vi "TDMS_Waveform to file.vi"(0 "Base path":path, 1 "Group Name":string="A", 2 "Interval":T1=enum."Daily", 3 "UTC Time FPGA":u64[](array[numeric]), 5 "Measurement":string, 9 "element":waveform(dbl)[](array[waveform]), 11 "error in (no error)":errorcluster, 12 "Channel Names":string[](array[string]), 13 "property values":variant[](array[variant]), 14 "UTC Time SC":u64[](array[numeric])) -> (4 "file out":refnum<k34>, 15 "error out":errorcluster)   [LabVIEW 2019]
uses:
  Globals and Definitions/Enum_FileNewInterval.ctl
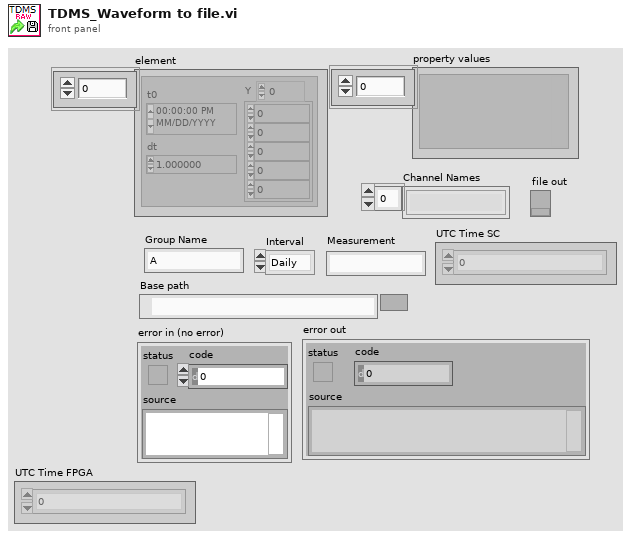
[diagram p1: front panel]
types:
  T1 = typedef "Enum_FileNewInterval.ctl" = enum16{"10 Min", "Hourly", "Daily", "Weekly", "Monthly"}
  T2 = enum16{"open", "open or create", "create or replace", "create", "open (read-only)"}
  T3 = typedef "LVDateTimeRec.ctl" = cluster{"fractional second":dbl, "second":i32, "minute":i32, "hour":i32, "day of month":i32, "month":i32, "year":i32, "day of week":i32, "day of year":i32, "DST":i32}
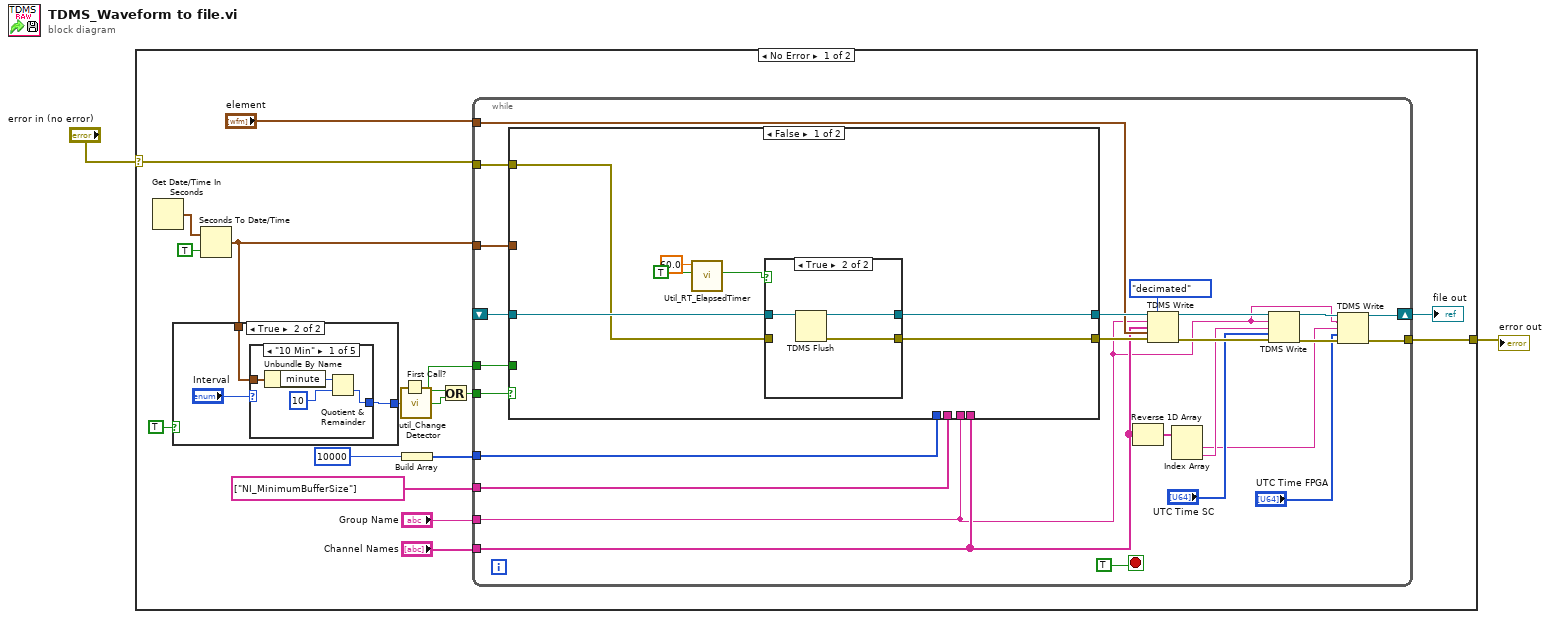
[diagram p0: block diagram]
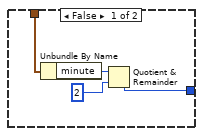
[diagram p2: hidden frame]
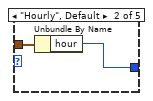
[diagram p3: hidden frame]
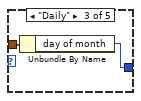
[diagram p4: hidden frame]
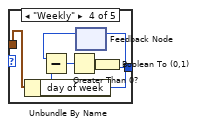
[diagram p5: hidden frame]
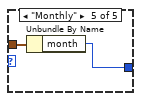
[diagram p6: hidden frame]
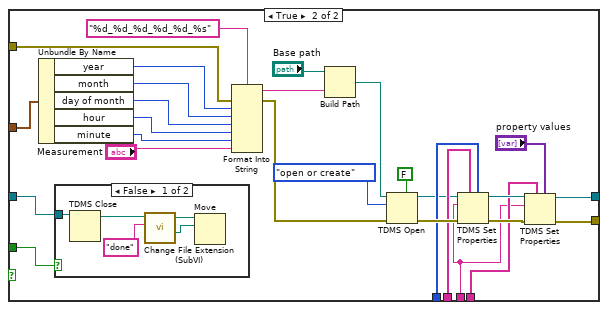
[diagram p8: hidden frame]
diagram:
  n1 = case shown="No Error" "error in (no error)" {
    selector: "error in (no error)" -> [w5 w113]
    tunnel: [w17 w113] -> w2
    frame No Error {
      n2 = Get Date/Time In Seconds() -> (seconds since 1Jan1904=w10:timestamp)
      n3 = Seconds To Date/Time(time stamp (now)=w10, to UTC (F)=TRUE) -> (date time rec=w9:T3)
      n4 = case shown="True" TRUE {
        tunnel: w9 -> [w21 w25]
        tunnel: [w20 w24] -> w7
        frame False {
          n5 = Unbundle By Name(w21) -> ("minute"=w23:i32)
          n6 = Quotient & Remainder(x=w23, y=2) -> (floor(x/y)=w20:i32)  [unwired: 1 out]
        }
        frame True {
          n7 = case shown="\"10 Min\"" "Interval" {
            tunnel: w25 -> [w30 w32 w34 w40 w42]
            tunnel: [w27 w31 w33 w35 w41] -> w24
            frame "10 Min" {
              n8 = Unbundle By Name(w30) -> ("minute"=w29:i32)
              n9 = Quotient & Remainder(x=w29, y=10) -> (floor(x/y)=w27:i32)  [unwired: 1 out]
            }
            frame "Hourly", Default {
              n10 = Unbundle By Name(w32) -> ("hour"=w31:i32)
            }
            frame "Daily" {
              n11 = Unbundle By Name(w34) -> ("day of month"=w33:i32)
            }
            frame "Weekly" {
              n12 = Unbundle By Name(w40) -> ("day of week"=w38:i32)
              n13 = feedback-in #1(w38) -> ()
              n14 = feedback #1() -> (w39:i32)  [unwired: 1 in]
              n15 = Subtract(x=w39, y=w38) -> (x-y=w37:i32)
              n16 = Greater Than 0?(x=w37) -> (x > 0?=w36:bool)
              n17 = Boolean To (0,1)(Boolean=w36) -> (0, 1=w35:i16)
            }
            frame "Monthly" {
              n18 = Unbundle By Name(w42) -> ("month"=w41:i32)
            }
          }
        }
      }
      n19 = First Call?() -> (First Call?: T/F=w18:bool)
      n20 = call "util_Change Detector.vi"("value"=w7) -> ("changed?"=w8:bool)
      n21 = Build Array(10000) -> (w15:i32[])
      n22 = Or(x=w18, y=w8) -> (x .or. y?=w19:bool)
      n23 = while {
        tunnel: w19 -> [w67]
        shift-right: [w48] -> w3
        shift-left: _ -> [w66]
        tunnel: w18 -> [w65]
        tunnel: [w47] -> w17
        tunnel: w9 -> [w62]
        tunnel: w15 -> [w61]
        tunnel: string[] ["NI_MinimumBufferSize"] ("Channel Names") -> [w60]
        tunnel: "Group Name" -> [w45]
        tunnel: "Channel Names" -> [w51]
        tunnel: "element" -> [w56]
        tunnel: w5 -> [w57]
        stop <- TRUE stop-if-true
        n24 = case shown="False" w67 {
          tunnel: w66 -> [w74 w104]
          tunnel: w65 -> [_ w105]
          tunnel: [w71 w85] -> w59
          tunnel: w62 -> [_ w102]
          tunnel: [w69 w87] -> w58
          tunnel: w61 -> [_ w100]
          tunnel: w60 -> [_ w99]
          tunnel: w45 -> [_ w82]
          tunnel: w51 -> [_ w83]
          tunnel: w57 -> [w68 w89]
          frame False {
            n25 = call "Util_RT_ElapsedTimer.vi"("Auto Reset"=TRUE, "Target Time (s)"=60.0) -> ("Target\nReached"=w70:bool)  [unwired: 8 in, 1 out]
            n26 = case shown="True" w70 {
              tunnel: w74 -> [w76 w79]
              tunnel: [w76 w78] -> w69
              tunnel: [w75 w77] -> w71
              tunnel: w68 -> [w75 _]
              frame False {
              }
              frame True {
                n27 = TDMS Flush(7:w79) -> (0:w77:errorcluster, 3:w78:refnum<k34>)  [unwired: 1 in]
              }
            }
          }
          frame True {
            n28 = Unbundle By Name(w102) -> ("year"=w97:i32, "month"=w96:i32, "day of month"=w95:i32, "hour"=w94:i32, "minute"=w93:i32)
            n29 = case shown="False" w105 {
              tunnel: w104 -> [w112 _]
              frame False {
                n30 = TDMS Close(11:w112) -> (3:w111:path)  [unwired: 1 in, 1 out]
                n31 = call "Change File Extension (SubVI).vi"("New Extension"="done", "appended path"=w111) -> ("New file path"=w108:path, "Original Path"=w110:path)  [unwired: 7 in, 1 out]
                n32 = Move(source path=w110, 10:w108) -> ()  [unwired: 3 in, 3 out]
              }
              frame True {
              }
            }
            n33 = Format Into String(format string="%d_%d_%d_%d_%d_%s", error in=w89, w97, w96, w95, w94, w93, "Measurement") -> (resulting string=w98:string, error out=w103:errorcluster)  [unwired: 1 in]
            n34 = Build Path(base path="Base path", name or relative path=w98) -> (appended path=w80:path)
            n35 = TDMS Open(5:FALSE ("create index file? (T)"), 8:w103, 10:T2."open or create" ("operation (0:open)"), 11:w80) -> (0:w101:errorcluster, 3:w91:refnum<k34>)  [unwired: 3 in]
            n36 = TDMS Set Properties(5:w100, 7:w99, 8:w101, 10:w82, 11:w91) -> (0:w86:errorcluster, 3:w88:refnum<k34>)  [unwired: 1 in, 2 out]
            n37 = TDMS Set Properties(5:"property values", 7:w83, 8:w86, 10:w82, 11:w88) -> (0:w85:errorcluster, 3:w87:refnum<k34>)  [unwired: 1 in, 2 out]
          }
        }
        n38 = Reverse 1D Array(array=w51) -> (reversed array=w52:string[])
        n39 = TDMS Write(0:w58, 1:enum16{"decimated", "interleaved"}."decimated" ("data layout (0:decimated)"), 5:w45, 7:w51, 9:w56, 11:w59) -> (4:w55:refnum<k34>, 15:w54:errorcluster)  [unwired: 2 out]
        n40 = Index Array(array=w52) -> (element #1=w44:string, element #2=w50:string)  [unwired: 2 in]
        n41 = TDMS Write(0:w55, 5:w45, 7:w50, 9:"UTC Time SC", 11:w54) -> (4:w49:refnum<k34>, 15:w46:errorcluster)  [unwired: 1 in, 2 out]
        n42 = TDMS Write(0:w49, 5:w45, 7:w44, 9:"UTC Time FPGA", 11:w46) -> (4:w48:refnum<k34>, 15:w47:errorcluster)  [unwired: 1 in, 2 out]
      }
      "file out" <- w3
    }
    frame Error {
    }
  }
  "error out" <- w2
